vi "Eject Coin.vi"(0 "reference in":refnum<class "No Coin State.lvclass">, 5 "error in (no error)":errorcluster) -> (14 "reference out":refnum<class "No Coin State.lvclass">, 19 "error out":errorcluster)   [LabVIEW 2013, in "No Coin State.lvclass"]
uses:
  No Coin State.lvclass
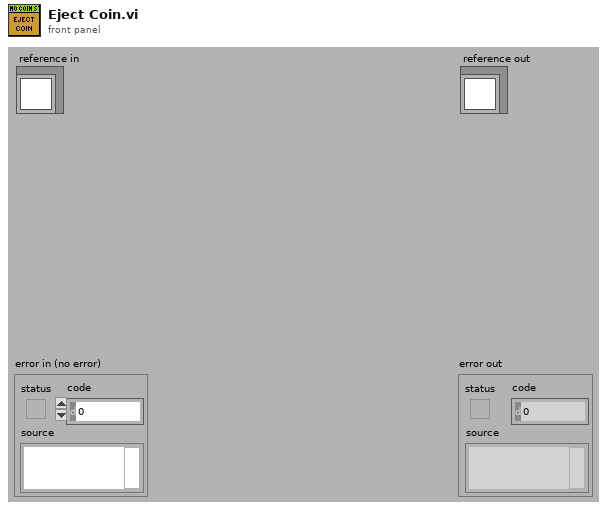
[diagram p1: front panel]
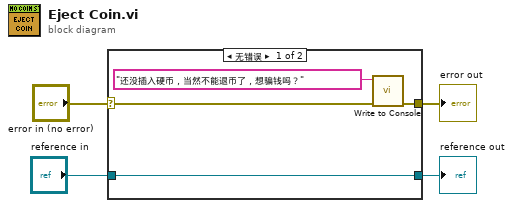
[diagram p0: block diagram]
diagram:
  n1 = case shown="无错误" "error in (no error)" {
    selector: "error in (no error)" -> [w7 w10]
    tunnel: [w5 w10] -> w3
    tunnel: [w8 w9] -> w1
    tunnel: "reference in" -> [w8 w9]
    frame No Error {
      n2 = call "Write to Console.vi"("error in (no error)"=w7, "Input"="还没插入硬币，当然不能退币了，想骗钱吗？") -> ("error out"=w5:errorcluster)  [unwired: 9 in]
    }
    frame Error {
    }
  }
  "error out" <- w3
  "reference out" <- w1
